vi "Automatic Teller Machinenew (ATM).vi"() -> ()   [LabVIEW 2013]
doc: "This VI is the simulation of control system of ATM.\nwhen the application starts-\n-User input,Enter button,Left & Right Menu,Left & Right button is disabled and welcome message is displayed on ATM message indicator.\n-When card is inserted in card simulator it enable the User input and Enter button.\n-User input ask for account no and verify this acc. no. If account exist it enable the Left & Right Menu,Left & Right button And message indicato display main menu message."
uses:
  ATM/USB Template (LV 8.6)/Automatic Teller Machine/Controls/ATM States.ctl
panel:
  out "index of element":i32
  in  "Enter":bool
  in  "User Input":string
  in  "Right Buttons":T1
  out "Right Menu":T2
  in  "Left Buttons":T1
  out "Left Menu":T2
  in  "Card Simulator":bool
  out "ATM Messages":string
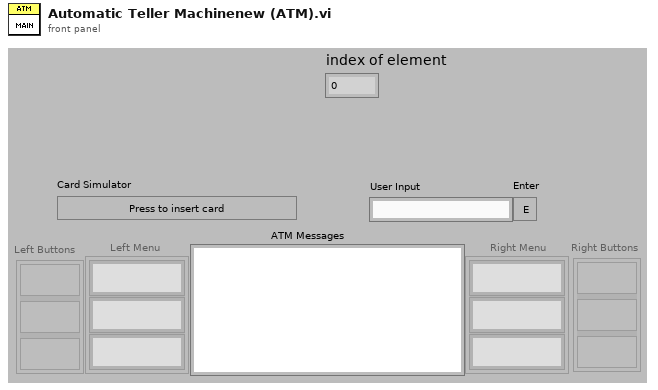
[diagram p1: front panel]
types:
  T1 = cluster{"Func Button":bool, "Func Button 2":bool, "Func Button 3":bool}
  T2 = cluster{"RFS String":string, "RFS String 2":string, "RFS String 3":string}
  T3 = typedef "ATM States.ctl" = enum16{"Initialize", "Card Simulator", "Insert ATM", "Deposit"}
  T4 = enum16{"Initialize", "Read", "Write", "Process", "Stop"}
  T5 = enum8{"Enabled", "Disabled", "Disabled and Grayed Out"}
  T6 = cluster{"Name":string, "Company":string, "Acc no.":string, "Balance":i32}[]
  T7 = cluster{"Name":string, "Company":string, "Acc no.":string, "Balance":i32}
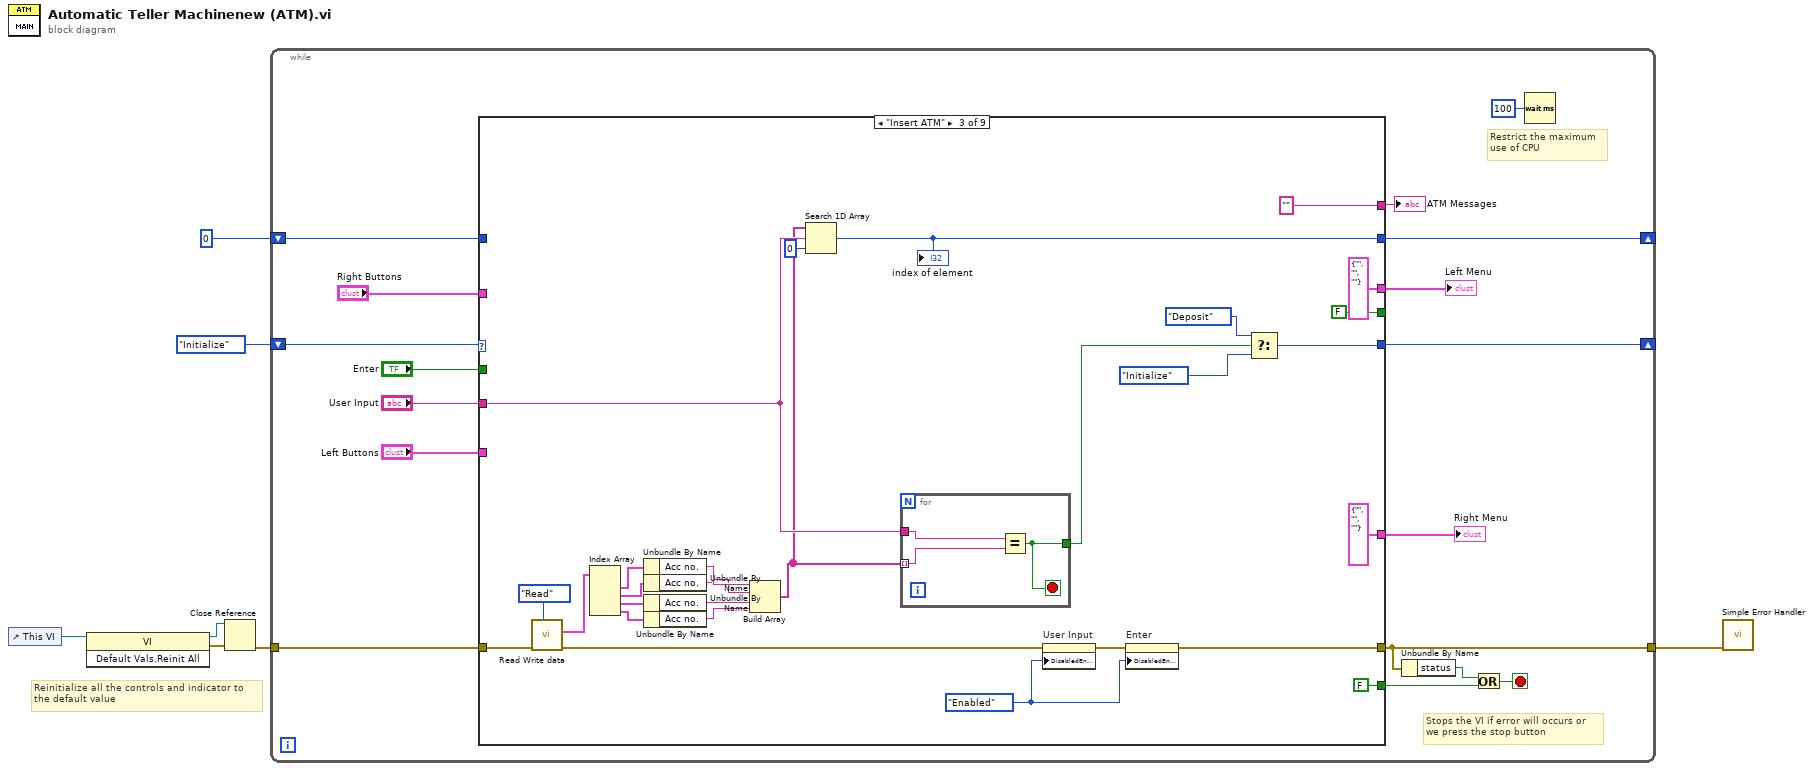
[diagram p0: block diagram]
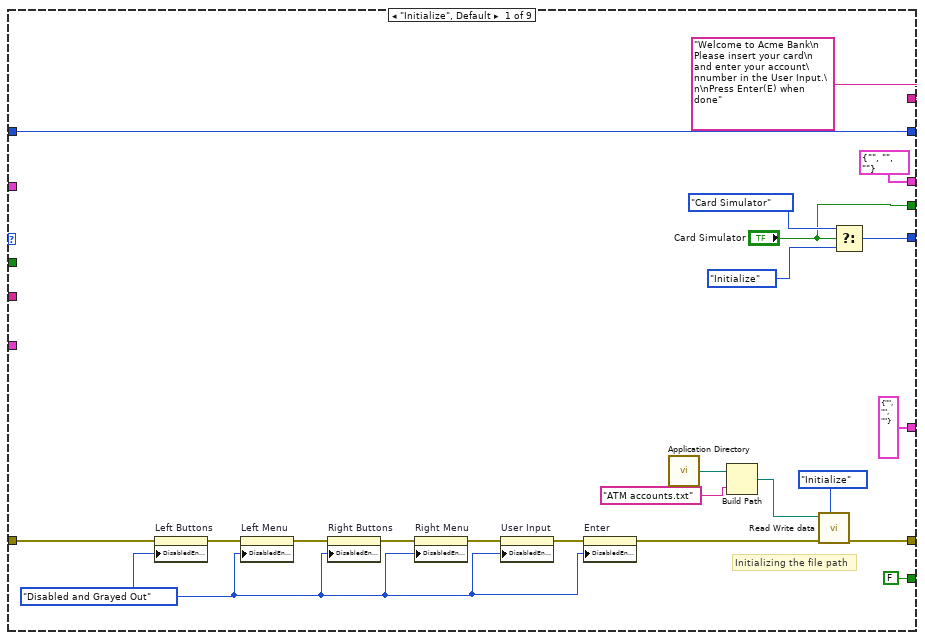
[diagram p2: hidden frame]
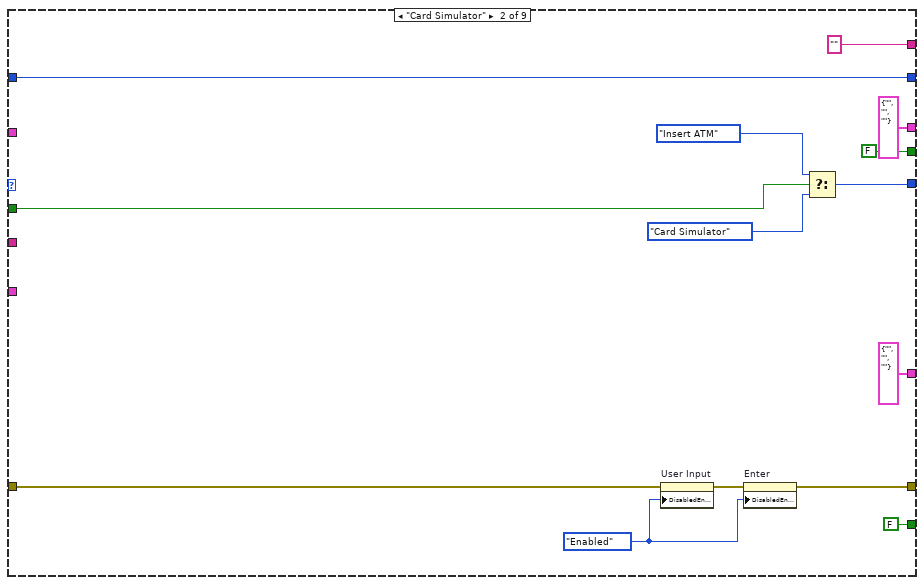
[diagram p3: hidden frame]
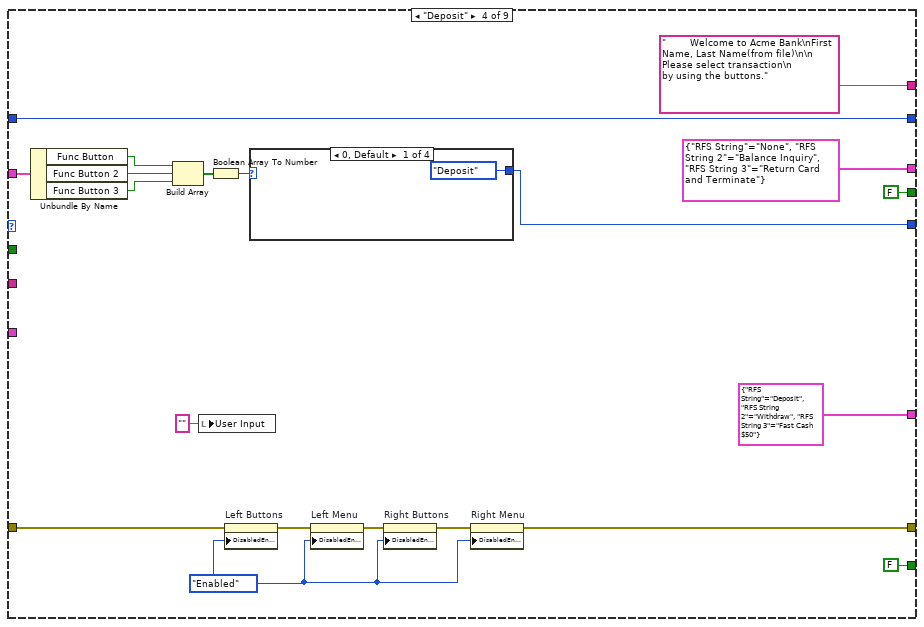
[diagram p4: hidden frame]
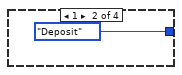
[diagram p5: hidden frame]
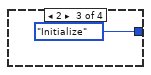
[diagram p6: hidden frame]
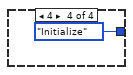
[diagram p7: hidden frame]
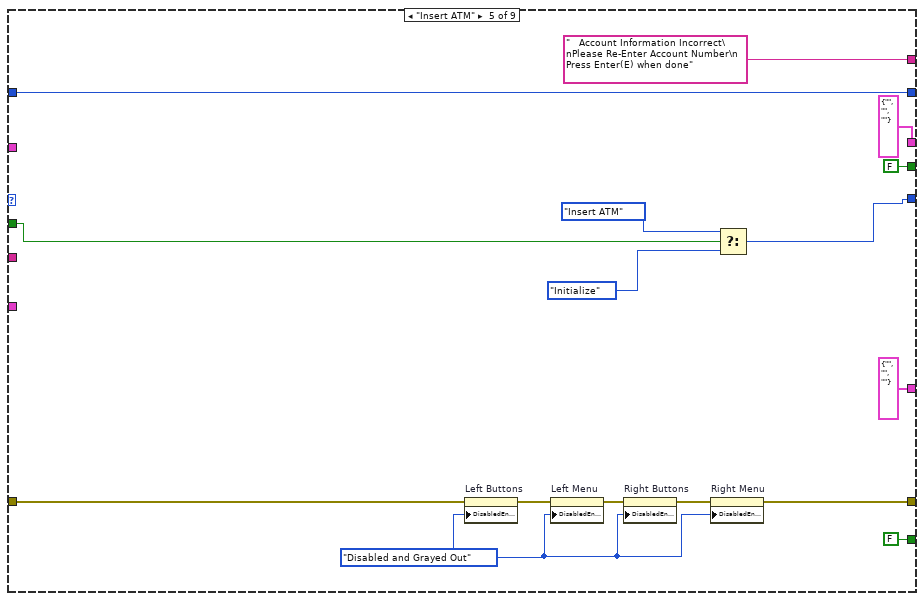
[diagram p8: hidden frame]
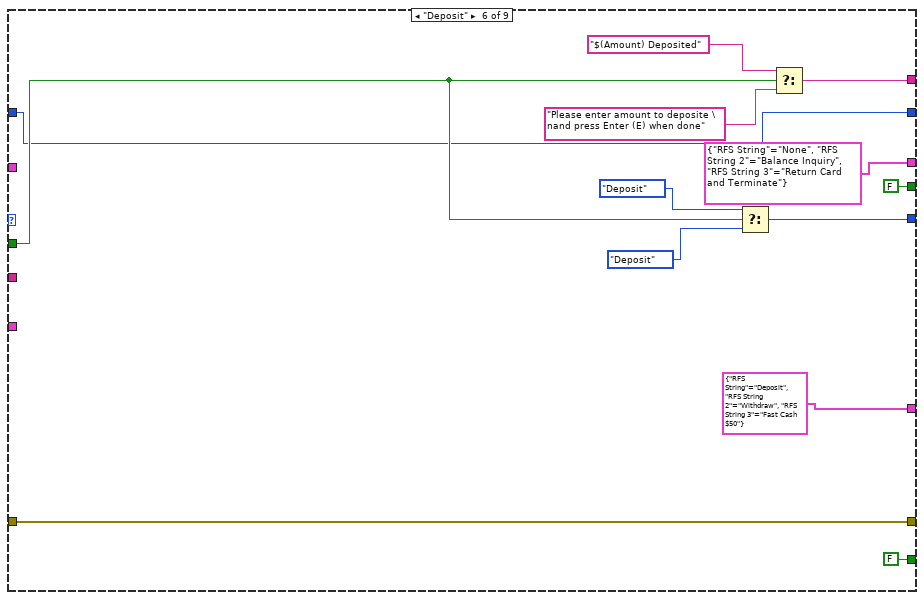
[diagram p9: hidden frame]
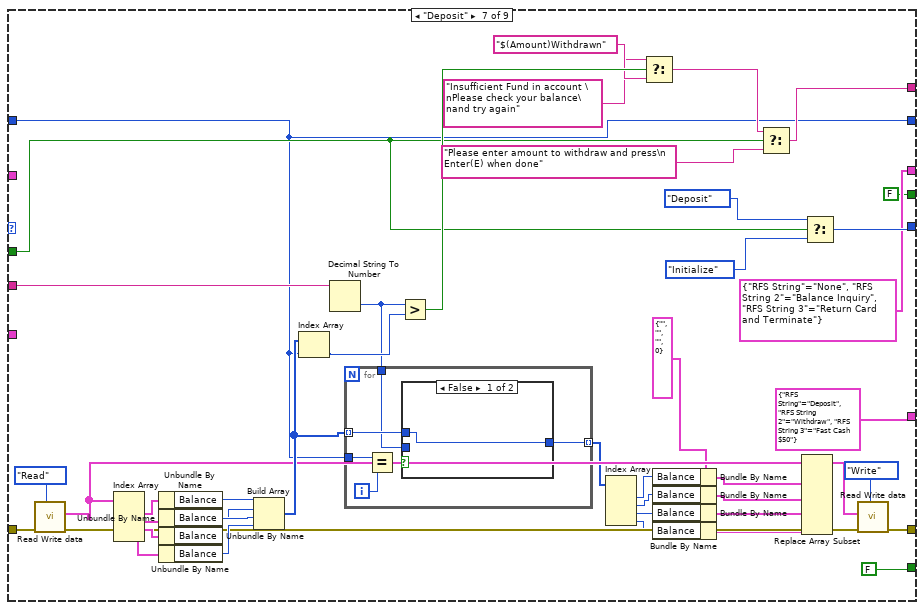
[diagram p10: hidden frame]
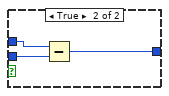
[diagram p11: hidden frame]
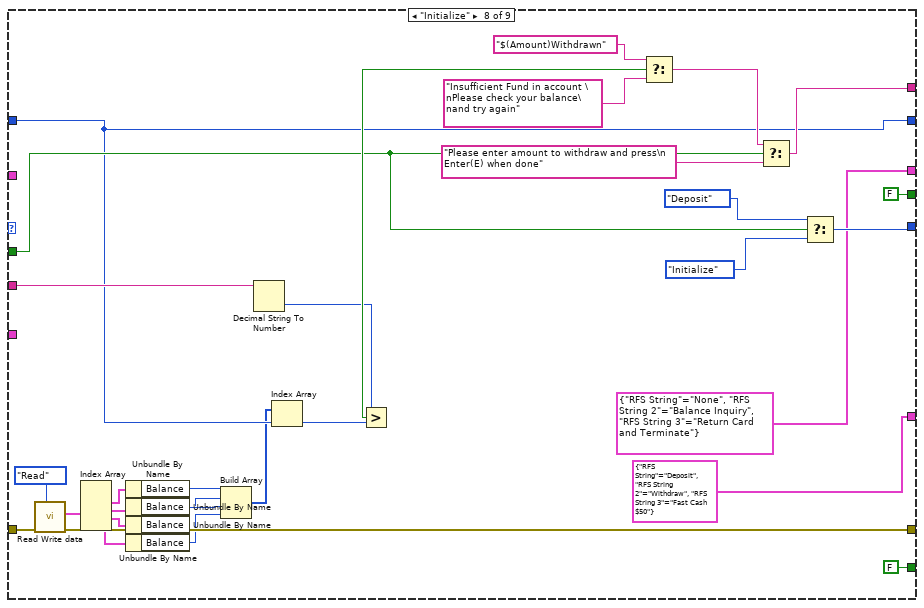
[diagram p12: hidden frame]
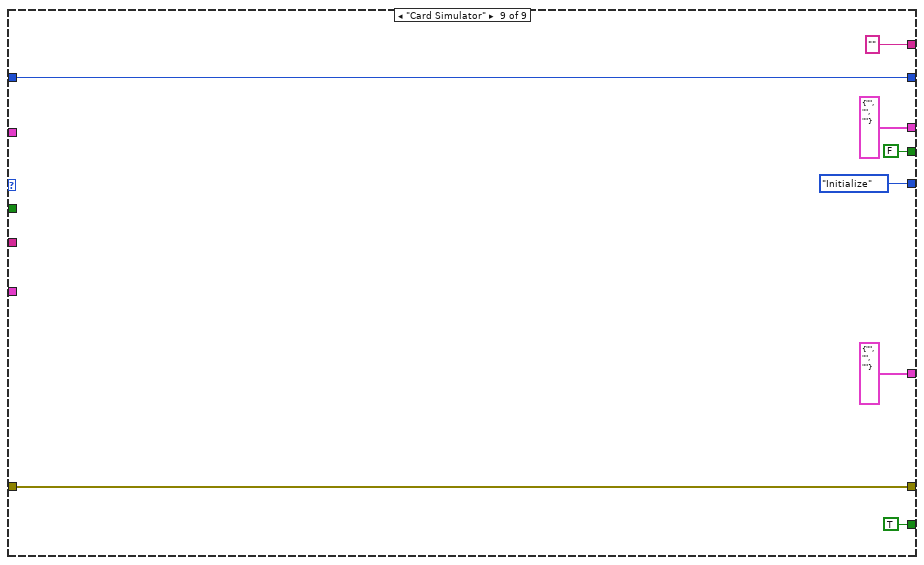
[diagram p13: hidden frame]
diagram:
  # "Reinitialize all the controls and indicator to \nthe default value"
  n1 = control-ref of="This VI"() -> (w6:refnum<vi>)
  n2 = invoke class="VI" method="Default Vals.Reinit All"(reference=w6) -> (reference out=w4:refnum<vi>, error out=w5:errorcluster)  [unwired: 2 in, 1 out]
  n3 = Close Reference(reference=w4, error in (no error)=w5) -> (error out=w3:errorcluster)
  n4 = while {
    tunnel: w3 -> [w23]
    tunnel: [w12] -> w2
    shift-right: [w8] -> _
    shift-left: ATM_States."Initialize" -> [w24]
    shift-right: [w18] -> _
    shift-left: 0 -> [w17]
    stop <- w11 stop-if-true
    # "Restrict the maximum\nuse of CPU"
    # "Stops the VI if error will occurs or \nwe press the stop button"
    n5 = case shown="\"Insert ATM\"" w24 {
      tunnel: w23 -> [w46 w56 w78 w95 w131 w132 w188 w229 w237]
      tunnel: [w35 w59 w87 w106 w125 w132 w161 w211 w237] -> w12
      tunnel: ["Welcome to Acme Bank\n Please insert your card\n and enter your account\nnumber in the User Input.\n\nPress Enter(E) when done" "" "" "        Welcome to Acme Bank\nFirst Name, Last Name(from file)\n\n         Please select transaction\n            by using the buttons." "   Account Information Incorrect\nPlease Re-Enter Account Number\n         Press Enter(E) when done" w142 w182 w223 ""] -> w22
      tunnel: "User Input" -> [_ _ w77 _ _ _ w180 w221 _]
      tunnel: [w30 w53 w79 w97 w118 w138 w177 w218 ATM_States."Initialize"] -> w8
      tunnel: [T2 {"RFS String"="", "RFS String 2"="", "RFS String 3"=""} ("Left Menu") T2 {"RFS String"="", "RFS String 2"="", "RFS String 3"=""} ("Left Menu") T2 {"RFS String"="", "RFS String 2"="", "RFS String 3"=""} ("Left Menu") T2 {"RFS String"="None", "RFS String 2"="Balance Inquiry", "RFS String 3"="Return Card and Terminate"} ("Left Menu") T2 {"RFS String"="", "RFS String 2"="", "RFS String 3"=""} ("Left Menu") T2 {"RFS String"="None", "RFS String 2"="Balance Inquiry", "RFS String 3"="Return Card and Terminate"} ("Left Menu") T2 {"RFS String"="None", "RFS String 2"="Balance Inquiry", "RFS String 3"="Return Card and Terminate"} ("Left Menu") T2 {"RFS String"="None", "RFS String 2"="Balance Inquiry", "RFS String 3"="Return Card and Terminate"} ("Left Menu") T2 {"RFS String"="", "RFS String 2"="", "RFS String 3"=""} ("Left Menu")] -> w20
      tunnel: [T2 {"RFS String"="", "RFS String 2"="", "RFS String 3"=""} ("Right Menu") T2 {"RFS String"="", "RFS String 2"="", "RFS String 3"=""} ("Right Menu") T2 {"RFS String"="", "RFS String 2"="", "RFS String 3"=""} ("Right Menu") T2 {"RFS String"="Deposit", "RFS String 2"="Withdraw", "RFS String 3"="Fast Cash $50"} ("Right Menu") T2 {"RFS String"="", "RFS String 2"="", "RFS String 3"=""} ("Right Menu") T2 {"RFS String"="Deposit", "RFS String 2"="Withdraw", "RFS String 3"="Fast Cash $50"} ("Right Menu") T2 {"RFS String"="Deposit", "RFS String 2"="Withdraw", "RFS String 3"="Fast Cash $50"} ("Right Menu") T2 {"RFS String"="Deposit", "RFS String 2"="Withdraw", "RFS String 3"="Fast Cash $50"} ("Right Menu") T2 {"RFS String"="", "RFS String 2"="", "RFS String 3"=""} ("Right Menu")] -> w19
      tunnel: "Right Buttons" -> [_ _ _ w103 _ _ _ _ _]
      tunnel: "Enter" -> [_ w52 _ _ w119 w139 w176 w217 _]
      tunnel: [w29 w51 w76 w94 w124 w137 w155 w216 w233] -> w18
      tunnel: w17 -> [w29 w51 _ w94 w124 w137 w155 w216 w233]
      tunnel: "Left Buttons" -> [_ _ _ _ _ _ _ _ _]
      tunnel: ["Card Simulator" FALSE ("Card Simulator") FALSE ("Card Simulator") FALSE ("Card Simulator") FALSE ("Card Simulator") FALSE ("Card Simulator") FALSE ("Card Simulator") FALSE ("Card Simulator") FALSE ("Card Simulator")] -> _
      tunnel: [FALSE FALSE FALSE FALSE FALSE FALSE FALSE FALSE TRUE] -> w9
      frame "Initialize", Default {
        w40 = T5."Disabled and Grayed Out" ("Disabled")
        # "Initializing the file path"
        n6 = property on="Left Buttons" class="Clust"(error in=w46, "DisabledEnum"=w40) -> (error out=w45:errorcluster)  [unwired: 1 in, 1 out]
        n7 = property on="Left Menu" class="Clust (strict)"(error in=w45, "DisabledEnum"=w40) -> (error out=w44:errorcluster)  [unwired: 1 in, 1 out]
        n8 = property on="Right Buttons" class="Clust"(error in=w44, "DisabledEnum"=w40) -> (error out=w43:errorcluster)  [unwired: 1 in, 1 out]
        n9 = property on="Right Menu" class="Clust (strict)"(error in=w43, "DisabledEnum"=w40) -> (error out=w42:errorcluster)  [unwired: 1 in, 1 out]
        n10 = property on="User Input" class="Str"(error in=w42, "DisabledEnum"=w40) -> (error out=w41:errorcluster)  [unwired: 1 in, 1 out]
        n11 = property on="Enter" class="Bool"(error in=w41, "DisabledEnum"=w40) -> (error out=w36:errorcluster)  [unwired: 1 in, 1 out]
        n12 = call <vilib>:"Application Directory.vi"() -> ("Application Directory"=w34:path)
        n13 = Build Path(base path=w34, name or relative path="ATM accounts.txt") -> (appended path=w32:path)
        n14 = call "Read Write data.vi"("Command"=T4."Initialize" ("Enum"), "error in (no error)"=w36, "file path"=w32) -> ("error IO"=w35:errorcluster)  [unwired: 7 in, 1 out]
        n15 = Select(t=ATM_States."Card Simulator", s="Card Simulator", f=ATM_States."Initialize") -> (s? t:f=w30:T3)
      }
      frame "Card Simulator" {
        w57 = T5."Enabled" ("Disabled")
        n16 = property on="User Input" class="Str"(error in=w56, "DisabledEnum"=w57) -> (error out=w60:errorcluster)  [unwired: 1 in, 1 out]
        n17 = property on="Enter" class="Bool"(error in=w60, "DisabledEnum"=w57) -> (error out=w59:errorcluster)  [unwired: 1 in, 1 out]
        n18 = Select(t=ATM_States."Insert ATM", s=w52, f=ATM_States."Card Simulator") -> (s? t:f=w53:T3)
      }
      frame "Insert ATM" {
        w85 = T5."Enabled" ("Disabled")
        n19 = call "Read Write data.vi"("Command"=T4."Read" ("Enum"), "error in (no error)"=w78) -> ("error IO"=w84:errorcluster, "Array out"=w71:T6)  [unwired: 8 in]
        n20 = Index Array(array=w71) -> (element #1=w70:T7, element #2=w69:T7, element #3=w68:T7, element #4=w67:T7)  [unwired: 4 in]
        n21 = Unbundle By Name(w70) -> ("Acc no."=w66:string)
        n22 = Unbundle By Name(w69) -> ("Acc no."=w65:string)
        n23 = Unbundle By Name(w68) -> ("Acc no."=w64:string)
        n24 = Unbundle By Name(w67) -> ("Acc no."=w63:string)
        n25 = Build Array(w66, w65, w64, w63) -> (w62:string[])
        n26 = Search 1D Array(1D array=w62, element=w77, start index (0)=0) -> (index of element=w76:i32)
        "index of element" <- w76
        n27 = for {
          tunnel: w77 -> [w91]
          tunnel: [w90] -> w82
          tunnel: w62 -> [w89] mode=indexing
          stop <- w90 stop-if-true
          n28 = Equal?(x=w91, y=w89) -> (x = y?=w90:bool)
        }
        n29 = property on="User Input" class="Str"(error in=w84, "DisabledEnum"=w85) -> (error out=w88:errorcluster)  [unwired: 1 in, 1 out]
        n30 = property on="Enter" class="Bool"(error in=w88, "DisabledEnum"=w85) -> (error out=w87:errorcluster)  [unwired: 1 in, 1 out]
        n31 = Select(t=ATM_States."Deposit", s=w82, f=ATM_States."Initialize") -> (s? t:f=w79:T3)
      }
      frame "Deposit" {
        w108 = T5."Enabled" ("Disabled")
        n32 = Unbundle By Name(w103) -> ("Func Button"=w102:bool, "Func Button 2"=w101:bool, "Func Button 3"=w100:bool)
        n33 = Build Array(w102, w101, w100) -> (w98:bool[])
        n34 = local write "User Input"("" ("User Input")) -> ()
        n35 = Boolean Array To Number(Boolean array=w98) -> (number=w99:u32)
        n36 = property on="Left Buttons" class="Clust"(error in=w95, "DisabledEnum"=w108) -> (error out=w111:errorcluster)  [unwired: 1 in, 1 out]
        n37 = case shown="0, Default" w99 {
          tunnel: [ATM_States."Deposit" ATM_States."Deposit" ATM_States."Initialize" ATM_States."Initialize"] -> w97
          frame 0, Default {
          }
          frame 1 {
          }
          frame 2 {
          }
          frame 4 {
          }
        }
        n38 = property on="Left Menu" class="Clust (strict)"(error in=w111, "DisabledEnum"=w108) -> (error out=w110:errorcluster)  [unwired: 1 in, 1 out]
        n39 = property on="Right Buttons" class="Clust"(error in=w110, "DisabledEnum"=w108) -> (error out=w109:errorcluster)  [unwired: 1 in, 1 out]
        n40 = property on="Right Menu" class="Clust (strict)"(error in=w109, "DisabledEnum"=w108) -> (error out=w106:errorcluster)  [unwired: 1 in, 1 out]
      }
      frame "Insert ATM" {
        w127 = T5."Disabled and Grayed Out" ("Disabled")
        n41 = property on="Left Buttons" class="Clust"(error in=w131, "DisabledEnum"=w127) -> (error out=w130:errorcluster)  [unwired: 1 in, 1 out]
        n42 = property on="Left Menu" class="Clust (strict)"(error in=w130, "DisabledEnum"=w127) -> (error out=w129:errorcluster)  [unwired: 1 in, 1 out]
        n43 = property on="Right Buttons" class="Clust"(error in=w129, "DisabledEnum"=w127) -> (error out=w128:errorcluster)  [unwired: 1 in, 1 out]
        n44 = property on="Right Menu" class="Clust (strict)"(error in=w128, "DisabledEnum"=w127) -> (error out=w125:errorcluster)  [unwired: 1 in, 1 out]
        n45 = Select(t=ATM_States."Insert ATM", s=w119, f=ATM_States."Initialize") -> (s? t:f=w118:T3)
      }
      frame "Deposit" {
        n46 = Select(t=ATM_States."Deposit", s=w139, f=ATM_States."Deposit") -> (s? t:f=w138:T3)
        n47 = Select(t="$(Amount) Deposited", s=w139, f="Please enter amount to deposite \nand press Enter (E) when done") -> (s? t:f=w142:string)
      }
      frame "Deposit" {
        w156 = T7 {"Name"="", "Company"="", "Acc no."="", "Balance"=0} ("data In")
        n48 = call "Read Write data.vi"("Command"=T4."Read" ("Enum"), "error in (no error)"=w188) -> ("error IO"=w162:errorcluster, "Array out"=w157:T6)  [unwired: 8 in]
        n49 = Index Array(array=w157) -> (element #1=w171:T7, element #2=w170:T7, element #3=w169:T7, element #4=w168:T7)  [unwired: 4 in]
        n50 = Unbundle By Name(w171) -> ("Balance"=w164:i32)
        n51 = Unbundle By Name(w170) -> ("Balance"=w165:i32)
        n52 = Unbundle By Name(w169) -> ("Balance"=w166:i32)
        n53 = Unbundle By Name(w168) -> ("Balance"=w167:i32)
        n54 = Build Array(w164, w165, w166, w167) -> (w159:i32[])
        n55 = Index Array(array=w159, index=w155) -> (element=w163:i32)
        n56 = Decimal String To Number(string=w180) -> (number=w158:i32)  [unwired: 2 in, 1 out]
        n57 = for {
          tunnel: w159 -> [w191] mode=indexing
          tunnel: w155 -> [w194]
          tunnel: w158 -> [w190]
          tunnel: [w189] -> w153 mode=indexing
          i -> [w193]
          n58 = Equal?(x=w194, y=w193) -> (x = y?=w192:bool)
          n59 = case shown="False" w192 {
            tunnel: w191 -> [w195 w198]
            tunnel: w190 -> [_ w197]
            tunnel: [w195 w196] -> w189
            frame False {
            }
            frame True {
              n60 = Subtract(x=w198, y=w197) -> (x-y=w196:i32)
            }
          }
        }
        n61 = Greater?(x=w158, y=w163) -> (0:w187:bool)
        n62 = Index Array(array=w153) -> (element #1=w152:i32, element #2=w151:i32, element #3=w150:i32, element #4=w149:i32)  [unwired: 4 in]
        n63 = Select(t="Insufficient Fund in account \nPlease check your balance\nand try again", s=w187, f="$(Amount)Withdrawn") -> (s? t:f=w185:string)
        n64 = Bundle By Name(cluster=w156, "Balance"=w152) -> (w148:T7)
        n65 = Bundle By Name(cluster=w156, "Balance"=w151) -> (w147:T7)
        n66 = Bundle By Name(cluster=w156, "Balance"=w150) -> (w146:T7)
        n67 = Bundle By Name(cluster=w156, "Balance"=w149) -> (w145:T7)
        n68 = Select(t=w185, s=w176, f="Please enter amount to withdraw and press\n                    Enter(E) when done") -> (s? t:f=w182:string)
        n69 = Replace Array Subset(array=w157, new element #1=w148, new element #2=w147, new element #3=w146, new element #4=w145) -> (w154:T6)  [unwired: 4 in]
        n70 = Select(t=ATM_States."Deposit", s=w176, f=ATM_States."Initialize") -> (s? t:f=w177:T3)
        n71 = call "Read Write data.vi"("Command"=T4."Write" ("Enum"), "error in (no error)"=w162, "Array in"=w154) -> ("error IO"=w161:errorcluster)  [unwired: 7 in, 1 out]
      }
      frame "Initialize" {
        n72 = call "Read Write data.vi"("Command"=T4."Read" ("Enum"), "error in (no error)"=w229) -> ("error IO"=w211:errorcluster, "Array out"=w202:T6)  [unwired: 8 in]
        n73 = Index Array(array=w202) -> (element #1=w210:T7, element #2=w209:T7, element #3=w208:T7, element #4=w207:T7)  [unwired: 4 in]
        n74 = Unbundle By Name(w210) -> ("Balance"=w203:i32)
        n75 = Unbundle By Name(w209) -> ("Balance"=w204:i32)
        n76 = Unbundle By Name(w208) -> ("Balance"=w205:i32)
        n77 = Unbundle By Name(w207) -> ("Balance"=w206:i32)
        n78 = Build Array(w203, w204, w205, w206) -> (w201:i32[])
        n79 = Decimal String To Number(string=w221) -> (number=w199:i32)  [unwired: 2 in, 1 out]
        n80 = Index Array(array=w201, index=w216) -> (element=w200:i32)
        n81 = Greater?(x=w199, y=w200) -> (0:w228:bool)
        n82 = Select(t="$(Amount)Withdrawn", s=w228, f="Insufficient Fund in account \nPlease check your balance\nand try again") -> (s? t:f=w226:string)
        n83 = Select(t=w226, s=w217, f="Please enter amount to withdraw and press\n                    Enter(E) when done") -> (s? t:f=w223:string)
        n84 = Select(t=ATM_States."Deposit", s=w217, f=ATM_States."Initialize") -> (s? t:f=w218:T3)
      }
      frame "Card Simulator" {
      }
    }
    "ATM Messages" <- w22
    "Left Menu" <- w20
    "Right Menu" <- w19
    n85 = Unbundle By Name(w12) -> ("status"=w10:bool)
    n86 = Or(x=w10, y=w9) -> (x .or. y?=w11:bool)
    n87 = Wait (ms)(milliseconds to wait=u32 100) -> ()  [unwired: 1 out]
  }
  n88 = call <vilib>:"Simple Error Handler.vi"("error in (no error)"=w2) -> ()  [unwired: 4 in, 5 out]
